vi "GE 5565PIORC.DMA.Enable.vi"(8 "error in (no error)":errorcluster, 10 "Enable DMA":bool, 11 "GE 5565PIORC in":refnum<class "GE 5565PIORC.lvclass">) -> (0 "error out":errorcluster, 3 "GE 5565PIORC out":refnum<class "GE 5565PIORC.lvclass">)   [LabVIEW 2016, in "GE 5565PIORC.lvclass"]
doc: "Enables or disables the ability to initiate DMA transfers."
uses:
  GE 5565PIORC.lvclass
  GE 5565PIORC.lvclass/GE 5565PIORC.ctl
  Properties/Registers/GE 5565PIORC.Registers.Local Configuration.Read.vi
  Properties/Registers/GE 5565PIORC.Registers.Local Configuration.Read (U8).vi
  Properties/Registers/GE 5565PIORC.Registers.Local Configuration.Write.vi
  Properties/Registers/GE 5565PIORC.Registers.Local Configuration.Write (U8).vi
  Properties/Registers/Bit Manipulation.Set Bit.vi
  Properties/Registers/Bit Manipulation.Set Bit (U8).vi
  Properties/Registers/GE 5565PIORC.Registers.Read.vi
  Properties/Registers/GE 5565PIORC.Registers.Read (U8).vi
  Properties/Registers/GE 5565PIORC.Registers.Write.vi
  Properties/Registers/GE 5565PIORC.Registers.Write (U8).vi
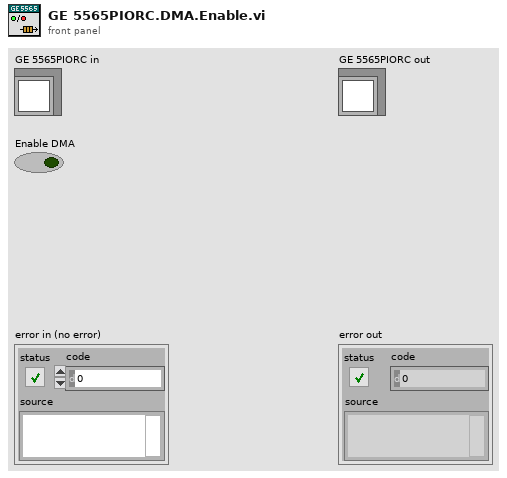
[diagram p1: front panel]
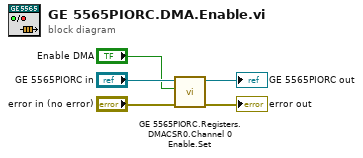
[diagram p0: block diagram]
diagram:
  n1 = call "GE 5565PIORC.Registers.DMACSR0.Channel 0 Enable.Set.vi"("error in (no error)"="error in (no error)", "Channel 0 Enable"="Enable DMA", "GE 5565PIORC in"="GE 5565PIORC in") -> ("error out"=→"error out":errorcluster, "GE 5565PIORC out"=→"GE 5565PIORC out":refnum<class "GE 5565PIORC.lvclass">)  [unwired: 7 in]
